vi "Do Something.vi"(8 "error in":errorcluster, 10 "Do Something Message":string) -> (0 "error out":errorcluster)   [LabVIEW 2019, in "My Singleton Module.lvlib"]
doc: "Send the Do something request to the Module's Main.vi.\n_____\nBased on DQMH Project Template 7.1.0.1447."
uses:
  My Singleton Module.lvlib
  Do Something Argument--cluster.ctl
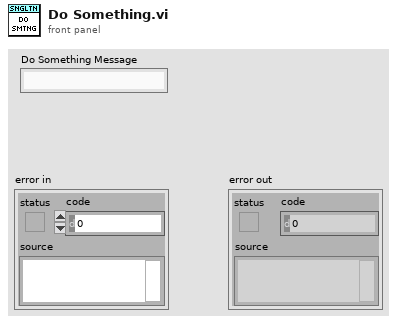
[diagram p1: front panel]
types:
  T1 = typedef "My Singleton Module.lvlib/Do Something Argument--cluster.ctl" = cluster{"Do Something Msg":string}
  T2 = typedef "My Singleton Module.lvlib/Request Events--cluster.ctl" = cluster{"Stop Module":refnum<user-event>, "Do Something":refnum<user-event>, "Do Something Else":refnum<user-event>, "Do Something Else and Wait for Reply":refnum<user-event>, "Show Panel":refnum<user-event>, "Hide Panel":refnum<user-event>, "Get Module Execution Status":refnum<user-event>, "Show Diagram":refnum<user-event>}
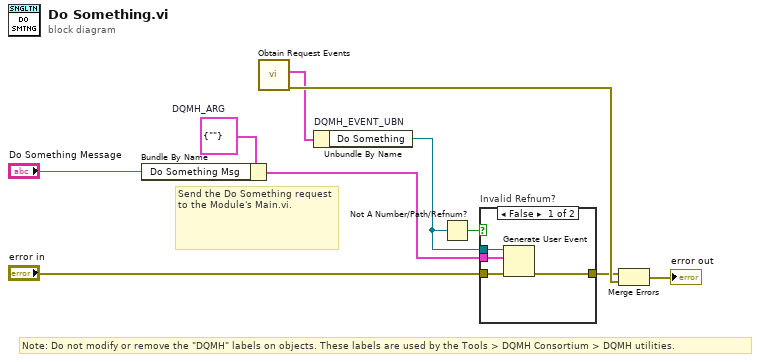
[diagram p0: block diagram]
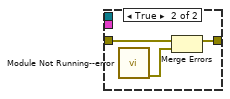
[diagram p2: hidden frame]
diagram:
  w4 = T1 {"Do Something Msg"=""}  # DQMH_ARG
  # "Note: Do not modify or remove the \"DQMH\" labels on objects. These labels are used by the Tools > DQMH Consortium > DQMH utilities."
  # "Send the Do Something request to the Module's Main.vi."
  n1 = Bundle By Name(cluster=w4, "Do Something Msg"="Do Something Message") -> (w3:T1)
  n2 = call "Obtain Request Events.vi"() -> ("error out"=w7:errorcluster, "My Singleton Module Request Events"=w5:T2)  [unwired: 10 in]
  n3 = Unbundle By Name "DQMH_EVENT_UBN"(w5) -> ("Do Something"=w2:refnum<user-event>)
  n4 = Not A Number/Path/Refnum?(number/path/refnum=w2) -> (NaN/Path/Refnum?=w1:bool)
  n5 = case "Invalid Refnum?" shown="False" w1 {
    tunnel: "error in" -> [w14 w15]
    tunnel: [w13 w16] -> w6
    tunnel: w3 -> [w12 _]
    tunnel: w2 -> [w11 _]
    frame False {
      n6 = Generate User Event(user event=w11, event data cluster=w12, error in=w14) -> (error out=w13:errorcluster)  [unwired: 1 in, 1 out]
    }
    frame True {
      n7 = call "Module Not Running--error.vi"() -> ("error out"=w17:errorcluster)  [unwired: 11 in]
      n8 = Merge Errors(w15, w17) -> (w16:errorcluster)
    }
  }
  n9 = Merge Errors(w6, w7) -> (→"error out":errorcluster)
